vi "Process Results.vi"(8 "error in (no error)":errorcluster, 9 "Measurement":variant, 10 "Test Limits":string[][](array[string]), 11 "Sub Test Name":string) -> (0 "error out":errorcluster, 3 "Results Data":string[](array[string]))   [LabVIEW 2024]
doc: "Generic results processor for numeric, boolean and string tests. Uses the limits file and sub test name to find the correct limits to be applied to the measurement."
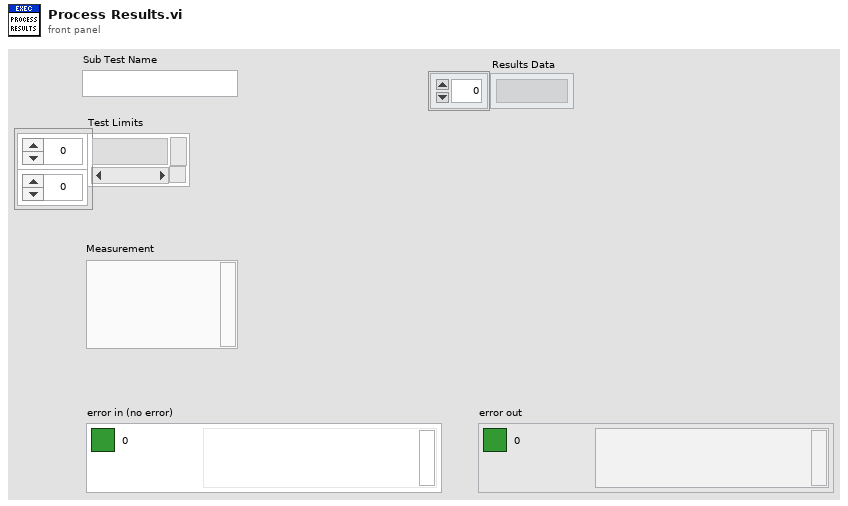
[diagram p1: front panel]
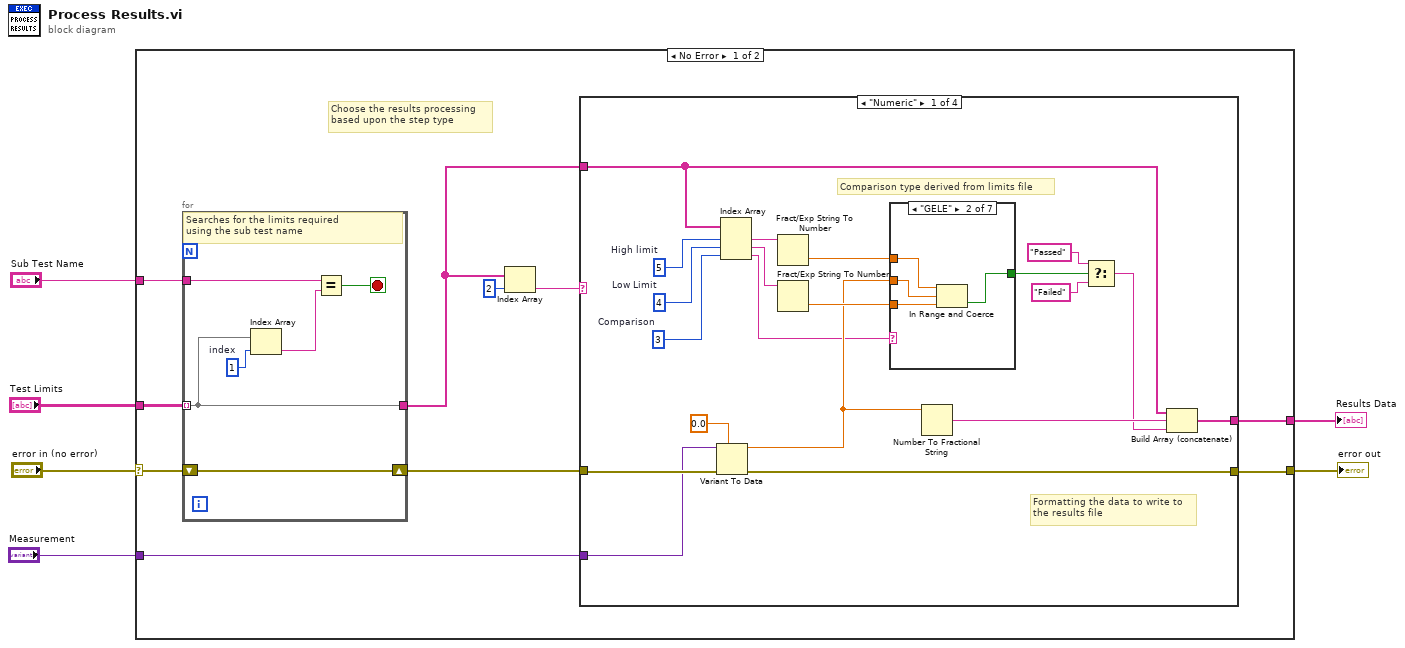
[diagram p0: block diagram]
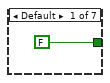
[diagram p2: hidden frame]
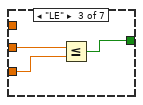
[diagram p3: hidden frame]
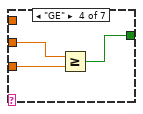
[diagram p4: hidden frame]
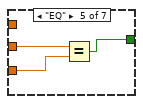
[diagram p5: hidden frame]
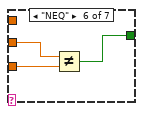
[diagram p6: hidden frame]
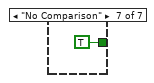
[diagram p7: hidden frame]
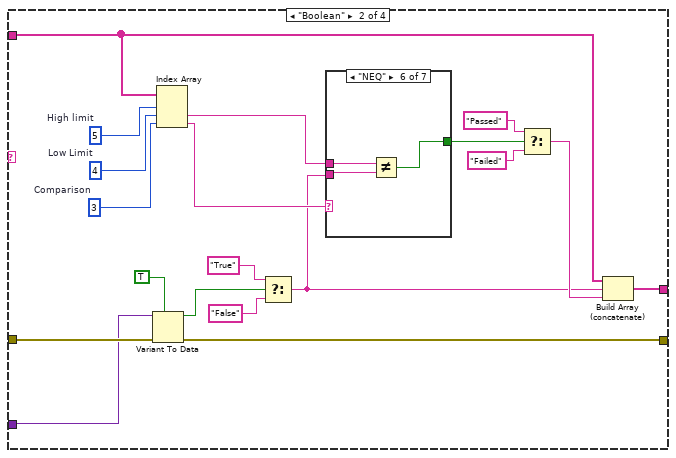
[diagram p8: hidden frame]
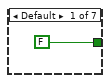
[diagram p9: hidden frame]
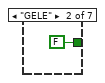
[diagram p10: hidden frame]
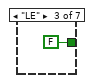
[diagram p11: hidden frame]
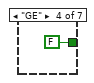
[diagram p12: hidden frame]
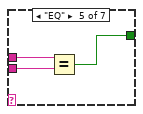
[diagram p13: hidden frame]
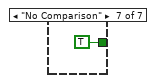
[diagram p14: hidden frame]
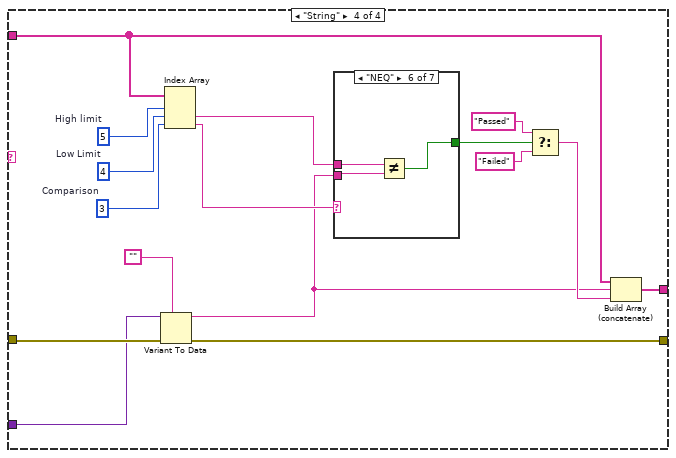
[diagram p16: hidden frame]
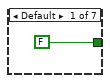
[diagram p17: hidden frame]
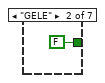
[diagram p18: hidden frame]
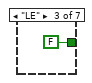
[diagram p19: hidden frame]
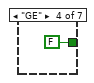
[diagram p20: hidden frame]
diagram:
  n1 = case shown="No Error" "error in (no error)" {
    selector: "error in (no error)" -> [w16 w121]
    tunnel: [w12 w121] -> w5
    tunnel: "Test Limits" -> [w15 _]
    tunnel: "Sub Test Name" -> [w14 _]
    tunnel: "Measurement" -> [w13 _]
    tunnel: [w11 string[] []] -> w1
    frame No Error {
      # "Choose the results processing \nbased upon the step type"
      n2 = for {
        tunnel: w15 -> [w18] mode=indexing
        tunnel: w14 -> [w21]
        tunnel: [w18] -> w10
        shift-right: [w17] -> w8
        shift-left: w16 -> [w17]
        stop <- w19 stop-if-true
        w22 = 1  # index
        # "Searches for the limits required\nusing the sub test name"
        n3 = Index Array(array=w18, index=w22) -> (element=w20:string)
        n4 = Equal?(x=w21, y=w20) -> (x = y?=w19:bool)
      }
      n5 = Index Array(array=w10, index=2) -> (element=w7:string)
      n6 = case shown="\"Numeric\"" w7 {
        tunnel: w13 -> [w41 w69 _ w97]
        tunnel: w8 -> [w42 w70 w92 w98]
        tunnel: w10 -> [w29 w71 w91 w99]
        tunnel: [w26 w67 w92 w96] -> w12
        tunnel: [w25 w61 w91 w95] -> w11
        frame "Numeric" {
          w23 = 3  # Comparison
          w35 = 4  # Low Limit
          w39 = 5  # High limit
          # "Formatting the data to write to\nthe results file"
          # "Comparison type derived from limits file"
          n7 = Variant To Data(error in=w42, type=0.0, Variant=w41) -> (data=w30:dbl, error out=w26:errorcluster)
          n8 = Index Array(array=w29, index #1=w39, index #2=w35, index #3=w23) -> (element #1=w38:string, element #2=w37:string, element #3=w24:string)
          n9 = Fract/Exp String To Number(string=w38) -> (number=w34:dbl)  [unwired: 3 in, 1 out]
          n10 = Fract/Exp String To Number(string=w37) -> (number=w33:dbl)  [unwired: 3 in, 1 out]
          n11 = case shown="\"GELE\"" w24 {
            tunnel: [FALSE w47 w48 w53 w56 w59 TRUE] -> w36
            tunnel: w34 -> [_ w46 _ _ _ _ _]
            tunnel: w33 -> [_ w45 w50 w51 w54 w57 _]
            tunnel: w30 -> [_ w44 w49 w52 w55 w58 _]
            frame Default {
            }
            frame "GELE" {
              n12 = In Range and Coerce(upper limit=w46, x=w44, lower limit=w45) -> (In Range?=w47:bool)  [unwired: 1 out]
            }
            frame "LE" {
              n13 = Less Or Equal?(x=w49, y=w50) -> (x <= y?=w48:bool)
            }
            frame "GE" {
              n14 = Greater Or Equal?(x=w52, y=w51) -> (x >= y?=w53:bool)
            }
            frame "EQ" {
              n15 = Equal?(x=w55, y=w54) -> (x = y?=w56:bool)
            }
            frame "NEQ" {
              n16 = Not Equal?(x=w58, y=w57) -> (x != y?=w59:bool)
            }
            frame "No Comparison" {
            }
          }
          n17 = Number To Fractional String(number=w30) -> (F-format string=w28:string)  [unwired: 3 in]
          n18 = Select(t="Passed", s=w36, f="Failed") -> (s? t:f=w27:string)
          n19 = Build Array (concatenate)(w29, w28, w27) -> (w25:string[])
        }
        frame "Boolean" {
          w74 = 3  # Comparison
          w75 = 4  # Low Limit
          w76 = 5  # High limit
          n20 = Variant To Data(error in=w70, type=TRUE, Variant=w69) -> (data=w66:bool, error out=w67:errorcluster)
          n21 = Index Array(array=w71, index #1=w76, index #2=w75, index #3=w74) -> (element #2=w63:string, element #3=w79:string)  [unwired: 1 out]
          n22 = Select(t="True", s=w66, f="False") -> (s? t:f=w62:string)
          n23 = case shown="\"NEQ\"" w79 {
            tunnel: [FALSE FALSE FALSE FALSE w86 w89 TRUE] -> w77
            tunnel: w62 -> [_ _ _ _ w84 w87 _]
            tunnel: w63 -> [_ _ _ _ w85 w88 _]
            frame Default {
            }
            frame "GELE" {
            }
            frame "LE" {
            }
            frame "GE" {
            }
            frame "EQ" {
              n24 = Equal?(x=w85, y=w84) -> (x = y?=w86:bool)
            }
            frame "NEQ" {
              n25 = Not Equal?(x=w88, y=w87) -> (x != y?=w89:bool)
            }
            frame "No Comparison" {
            }
          }
          n26 = Select(t="Passed", s=w77, f="Failed") -> (s? t:f=w78:string)
          n27 = Build Array (concatenate)(w71, w62, w78) -> (w61:string[])
        }
        frame "\u0000", Default {
        }
        frame "String" {
          w103 = 3  # Comparison
          w104 = 4  # Low Limit
          w105 = 5  # High limit
          n28 = Variant To Data(error in=w98, type="", Variant=w97) -> (data=w93:string, error out=w96:errorcluster)
          n29 = Index Array(array=w99, index #1=w105, index #2=w104, index #3=w103) -> (element #2=w100:string, element #3=w108:string)  [unwired: 1 out]
          n30 = case shown="\"NEQ\"" w108 {
            tunnel: [FALSE FALSE FALSE FALSE w115 w118 TRUE] -> w106
            tunnel: w93 -> [_ _ _ _ w113 w116 _]
            tunnel: w100 -> [_ _ _ _ w114 w117 _]
            frame Default {
            }
            frame "GELE" {
            }
            frame "LE" {
            }
            frame "GE" {
            }
            frame "EQ" {
              n31 = Equal?(x=w114, y=w113) -> (x = y?=w115:bool)
            }
            frame "NEQ" {
              n32 = Not Equal?(x=w117, y=w116) -> (x != y?=w118:bool)
            }
            frame "No Comparison" {
            }
          }
          n33 = Select(t="Passed", s=w106, f="Failed") -> (s? t:f=w107:string)
          n34 = Build Array (concatenate)(w99, w93, w107) -> (w95:string[])
        }
      }
    }
    frame Error {
    }
  }
  "error out" <- w5
  "Results Data" <- w1
